vi "When Write to Log.vi"(0 "error out":errorcluster, 11 "Log in":refnum<class "Mock Log.lvclass">) -> (3 "Log out":refnum<class "Mock Log.lvclass">)   [LabVIEW 2020, in "Mock Log.lvclass"]
uses:
  Mock Log.lvclass
  C:/Program Files (x86)/National Instruments/LabVIEW 2020/vi.lib/Astemes/LMock/Mock.lvclass
  <vilib>/Astemes/LMock/Mock.lvclass
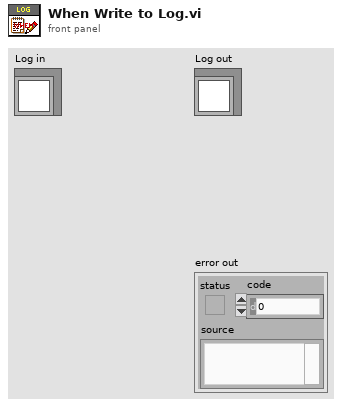
[diagram p1: front panel]
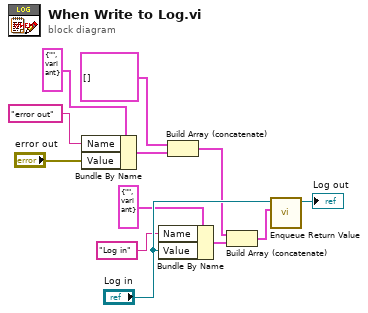
[diagram p0: block diagram]
diagram:
  n1 = Bundle By Name(cluster=cluster{"Name":string, "Value":variant} {"Name"="", "Value"=variant} ("element"), "Name"="error out", "Value"="error out") -> (w3:cluster{"Name":string, "Value":variant})
  n2 = Bundle By Name(cluster=cluster{"Name":string, "Value":variant} {"Name"="", "Value"=variant} ("element"), "Name"="Log in", "Value"="Log in") -> (w1:cluster{"Name":string, "Value":variant})
  n3 = Build Array (concatenate)(cluster{"Name":string, "Value":variant}[] [] ("Control Values"), w3) -> (w8:cluster{"Name":string, "Value":variant}[])
  n4 = Build Array (concatenate)(w8, w1) -> (w10:cluster{"Name":string, "Value":variant}[])
  n5 = call <vilib>:"Enqueue Return Value.vi"("Indicator Values"=w10, "Mock In"="Log in") -> ("Mock Out"=→"Log out":refnum<class "Mock Log.lvclass">)  [unwired: 8 in, 1 out]
